vi "FindMostRecentFile.vi"(8 "error in":errorcluster, 11 "Folder Path In":path) -> (0 "error out":errorcluster, 3 "File Path Out":path)   [LabVIEW 2015]
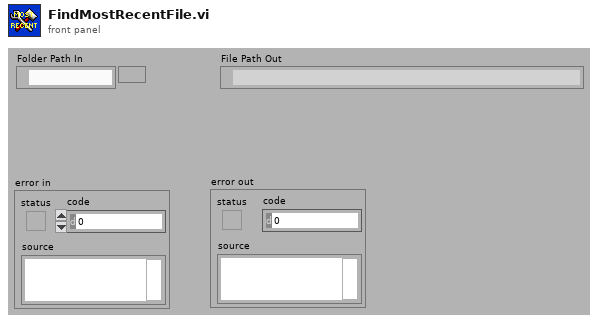
[diagram p1: front panel]
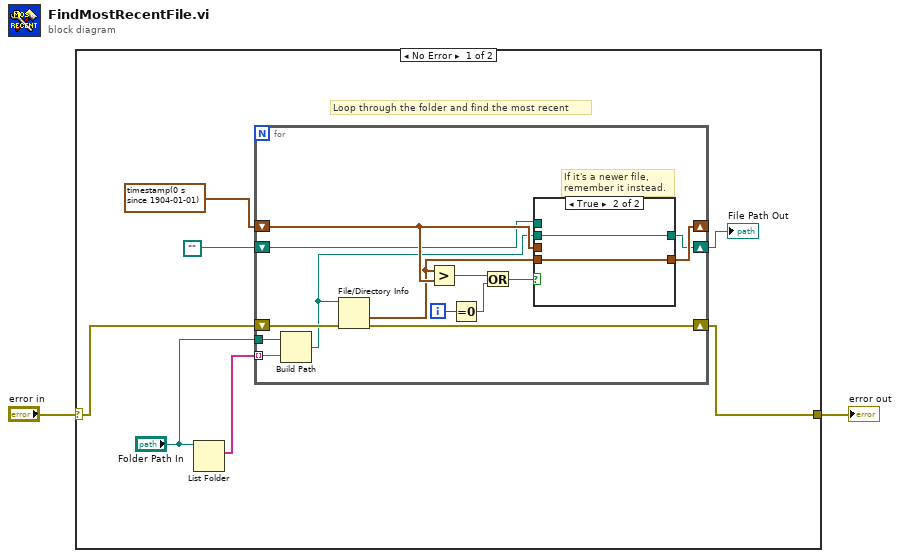
[diagram p0: block diagram]
diagram:
  n1 = case shown="No Error" "error in" {
    selector: "error in" -> [w5 w28]
    tunnel: [w9 w28] -> w2
    frame No Error {
      # "Loop through the folder and find the most recent"
      n2 = List Folder(path="Folder Path In") -> (filenames=w3:string[])  [unwired: 3 in, 3 out]
      n3 = for {
        shift-right: [w17] -> _
        shift-left: timestamp(0 s since 1904-01-01) ("last mod 2") -> [w18]
        shift-right: [w14] -> w8
        shift-left: path "" -> [w13]
        shift-right: [w12] -> w9
        shift-left: w5 -> [w23]
        tunnel: w3 -> [w11] mode=indexing
        tunnel: "Folder Path In" -> [w10]
        i -> [w19]
        # "If it's a newer file,\nremember it instead."
        n4 = Build Path(base path=w10, name or relative path=w11) -> (appended path=w15:path)
        n5 = File/Directory Info(path=w15, error in=w23) -> (last mod=w16:timestamp, error out=w12:errorcluster)  [unwired: 5 out]
        n6 = Greater?(x=w16, y=w18) -> (0:w21:bool)
        n7 = Equal To 0?(x=w19) -> (x = 0?=w20:bool)
        n8 = Or(x=w21, y=w20) -> (x .or. y?=w22:bool)
        n9 = case shown="True" w22 {
          tunnel: w18 -> [w25 _]
          tunnel: [w25 w27] -> w17
          tunnel: w16 -> [_ w27]
          tunnel: w15 -> [_ w26]
          tunnel: [w24 w26] -> w14
          tunnel: w13 -> [w24 _]
          frame False {
          }
          frame True {
          }
        }
      }
      "File Path Out" <- w8
    }
    frame Error {
    }
  }
  "error out" <- w2
